vi "PLC-PC.vi"() -> ()   [LabVIEW 2022 SP3]
uses:
  Labview/Globali.vi
panel:
  in  "DB10.DBW 254":u16
  in  "DB10.DBW 252":u16
  in  "DB10.DBW 250":u16
  in  "DB10.DBW 248":u16
  in  "DB10.DBW 246":u16
  in  "DB10.DBW 244":u16
  in  "DB10.DBW 242":u16
  in  "DB10.DBW 240":u16
  in  "DB10.DBW 238":u16
  in  "DB10.DBW 236":u16
  in  "DB10.DBW 234":u16
  in  "DB10.DBW 232":u16
  in  "DB10.DBW 230":u16
  in  "DB10.DBW 228":u16
  in  "DB10.DBW 226":u16
  in  "DB10.DBW 224":u16
  in  "DB10.DBW 222":u16
  in  "DB10.DBW 220":u16
  in  "DB10.DBW 218":u16
  in  "DB10.DBW 216":u16
  in  "DB10.DBW 214":u16
  in  "DB10.DBW 212":u16
  in  "DB10.DBW 210":u16
  in  "DB10.DBW 208":u16
  in  "DB10.DBW 206":u16
  in  "DB10.DBW 204":u16
  in  "DB10.DBW 202":u16
  in  "DB10.DBW 200":u16
  in  "DB10.DBW 198":u16
  in  "DB10.DBW 196":u16
  in  "DB10.DBW 194":u16
  in  "DB10.DBW 192":u16
  in  "DB10.DBW 190":u16
  in  "DB10.DBW 188":u16
  in  "DB10.DBW 186":u16
  in  "DB10.DBW 184":u16
  in  "DB10.DBW 182":u16
  in  "DB10.DBW 180":u16
  in  "DB10.DBW 178":u16
  in  "DB10.DBW 176":u16
  in  "DB10.DBW 174":u16
  in  "DB10.DBW 172":u16
  in  "DB10.DBW 170":u16
  in  "DB10.DBW 168":u16
  in  "DB10.DBW 166":u16
  in  "DB10.DBW 164":u16
  in  "DB10.DBW 162":u16
  in  "DB10.DBW 160":u16
  in  "DB10.DBW 158":u16
  in  "DB10.DBW 156":u16
  in  "DB10.DBW 154":u16
  in  "DB10.DBW 152":u16
  in  "DB10.DBW 150":u16
  in  "DB10.DBW 148":u16
  in  "DB10.DBW 146":u16
  in  "DB10.DBW 144":u16
  in  "DB10.DBW 142":u16
  in  "DB10.DBW 140":u16
  in  "DB10.DBW 138":u16
  in  "DB10.DBW 136":u16
  in  "DB10.DBW 134":u16
  in  "DB10.DBW 132":u16
  in  "DB10.DBW 130":u16
  in  "DB10.DBW 128":u16
  in  "DB10.DBW 126":u16
  in  "DB10.DBW 124":u16
  in  "DB10.DBW 122":u16
  in  "DB10.DBW 120":u16
  in  "DB10.DBW 118":u16
  in  "DB10.DBW 116":u16
  in  "DB10.DBW 114":u16
  in  "DB10.DBW 112":u16
  in  "DB10.DBW 110":u16
  in  "DB10.DBW 108":u16
  in  "DB10.DBW 106":u16
  in  "DB10.DBW 104":u16
  in  "DB10.DBW 102":u16
  in  "DB10.DBW 100":u16
  in  "DB10.DBW 98":u16
  in  "DB10.DBW 96":u16
  in  "DB10.DBW 94":u16
  in  "DB10.DBW 92":u16
  in  "DB10.DBW 90":u16
  in  "DB10.DBW 88":u16
  in  "DB10.DBW 86":u16
  in  "DB10.DBW 84":u16
  in  "DB10.DBW 82":u16
  in  "DB10.DBW 80":u16
  in  "DB10.DBW 78":u16
  in  "DB10.DBW 76":u16
  in  "DB10.DBW 74":u16
  in  "DB10.DBW 72":u16
  in  "DB10.DBW 70":u16
  in  "DB10.DBW 68":u16
  in  "DB10.DBW 66":u16
  in  "DB10.DBW 64":u16
  in  "DB10.DBW 62":u16
  in  "DB10.DBW 60":u16
  in  "DB10.DBW 58":u16
  in  "DB10.DBW 56":u16
  in  "DB10.DBW 54":u16
  in  "DB10.DBW 52":u16
  in  "DB10.DBW 50":u16
  in  "DB10.DBW 48":u16
  in  "DB10.DBW 46":u16
  in  "DB10.DBW 44":u16
  in  "DB10.DBW 42":u16
  in  "DB10.DBW 40":u16
  in  "DB10.DBW 38":u16
  in  "DB10.DBW 36":u16
  in  "DB10.DBW 34":u16
  in  "DB10.DBW 32":u16
  in  "DB10.DBW 30":u16
  in  "DB10.DBW 28":u16
  in  "DB10.DBW 26":u16
  in  "DB10.DBW 24":u16
  in  "DB10.DBW 22":u16
  in  "DB10.DBW 20":u16
  in  "DB10.DBW 18":u16
  in  "DB10.DBW 16":u16
  in  "DB10.DBW 14":u16
  in  "DB10.DBW 12":u16
  in  "DB10.DBW 10":u16
  in  "DB10.DBW 8":u16
  in  "DB10.DBW 6":u16
  in  "DB10.DBW 4":u16
  in  "DB10.DBW 2":u16
  in  "DB10.DBW 0":u16
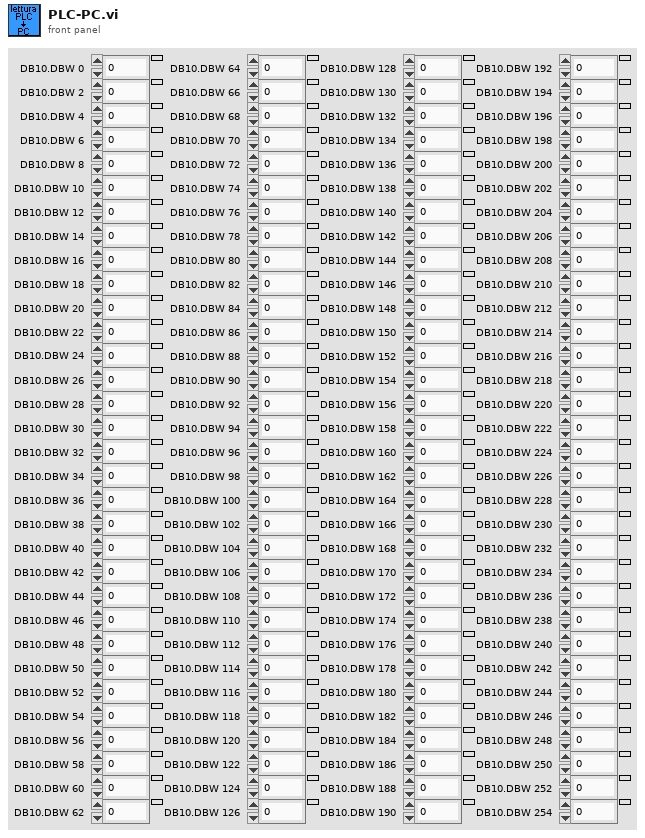
[diagram p1: front panel]
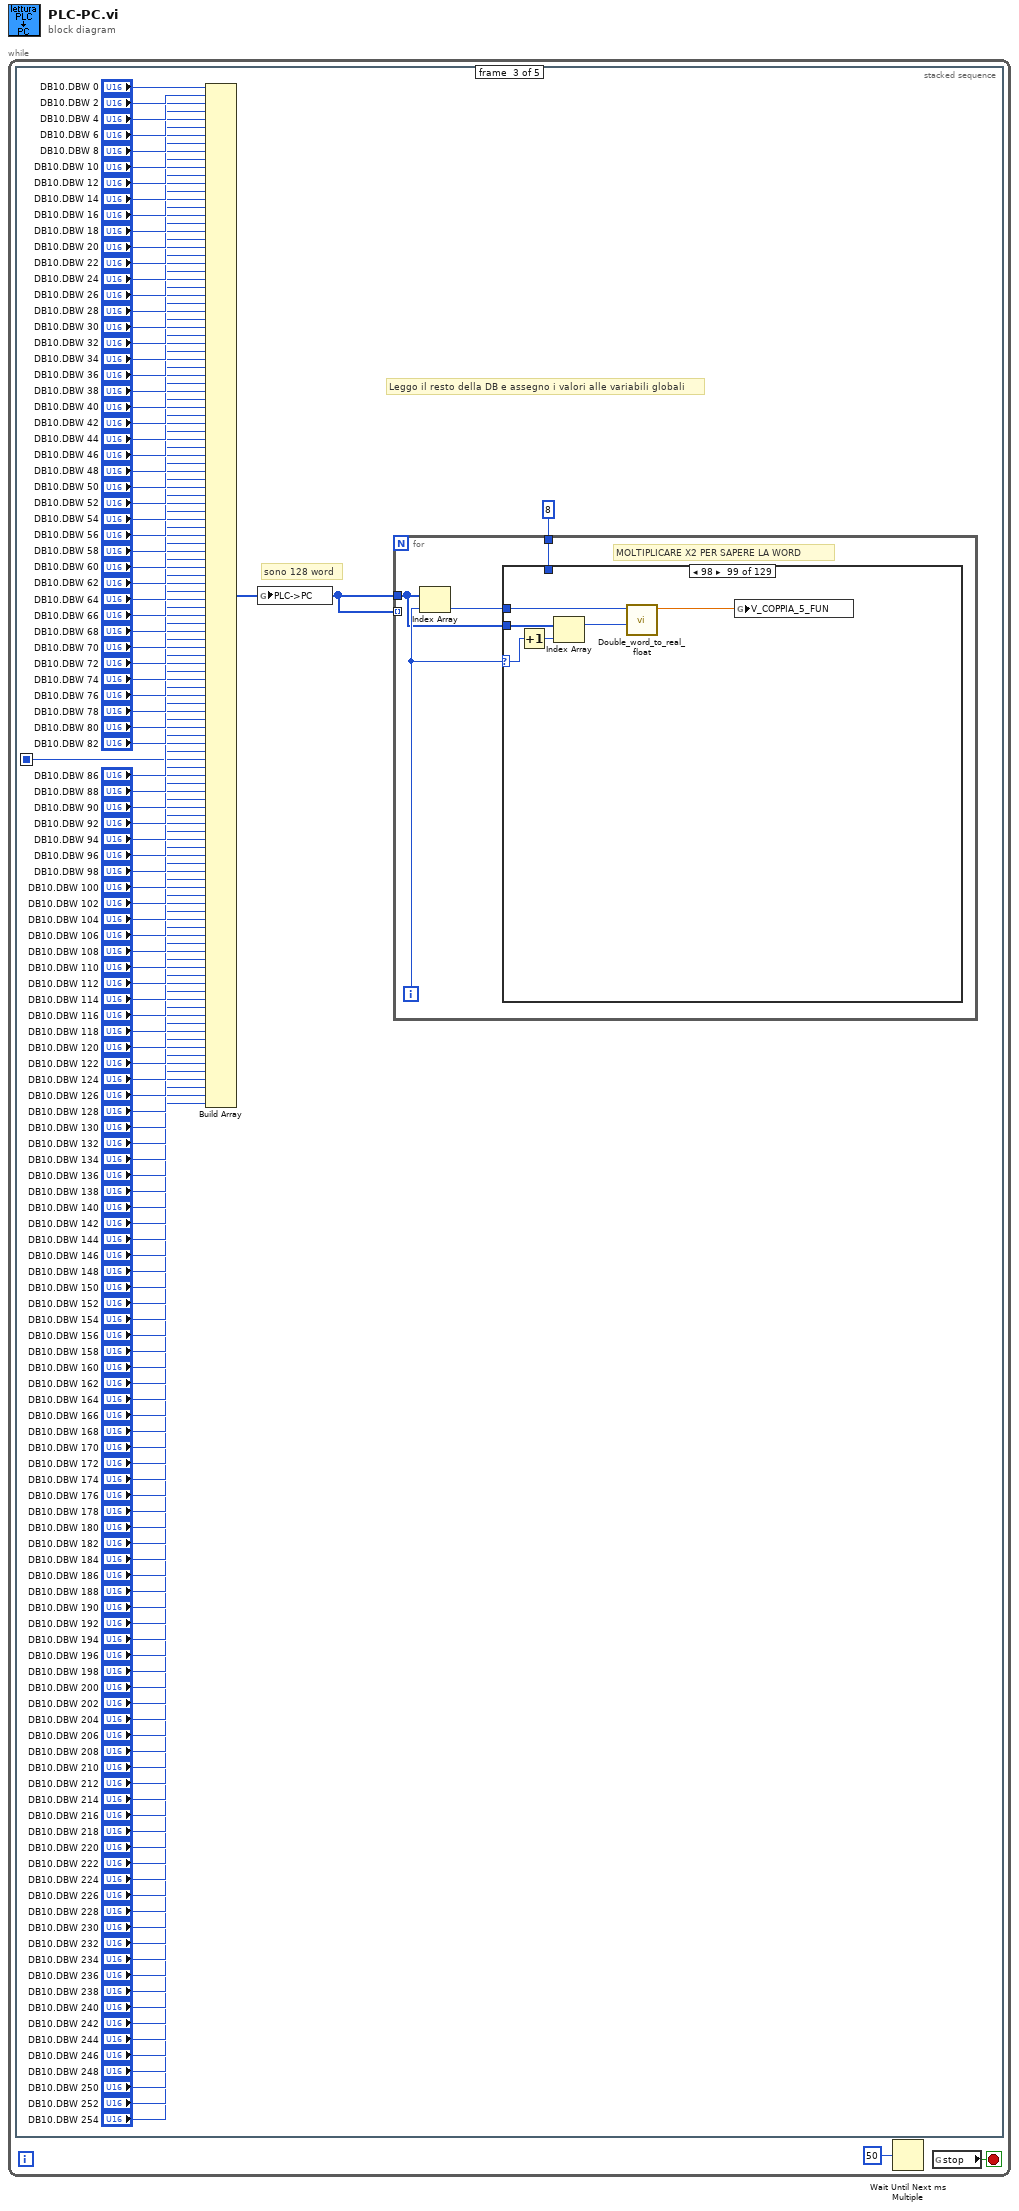
[diagram p0: block diagram]
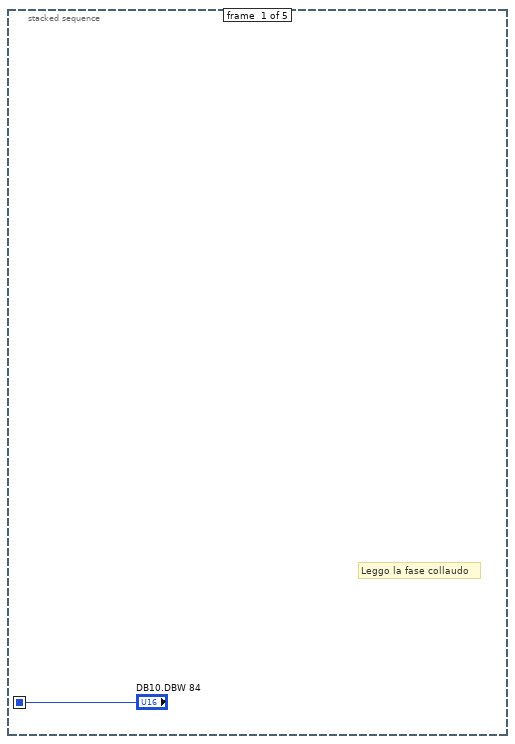
[diagram p2: hidden frame]
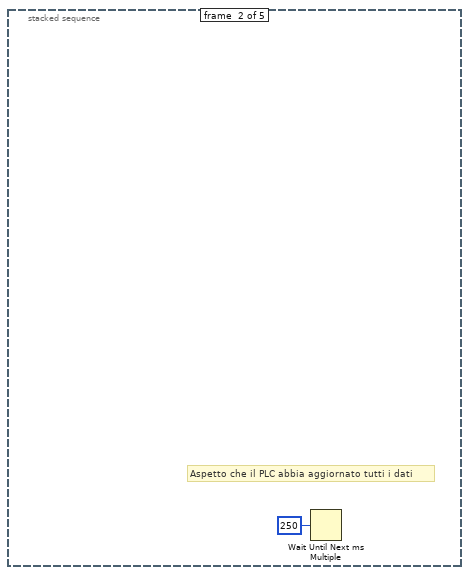
[diagram p3: hidden frame]
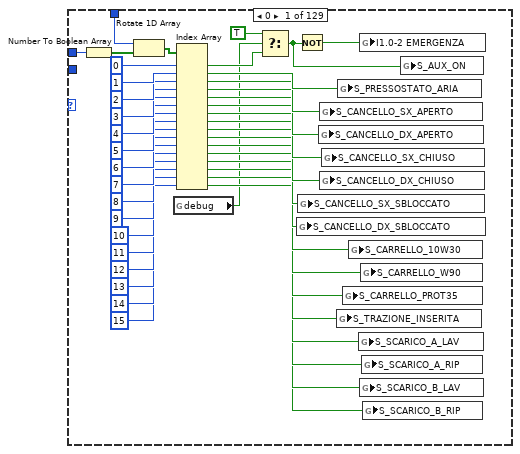
[diagram p4: hidden frame]
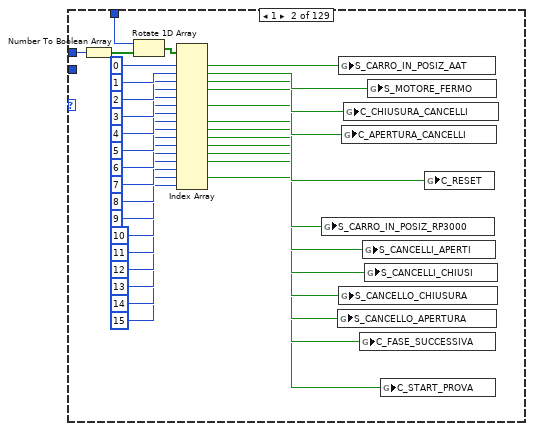
[diagram p5: hidden frame]
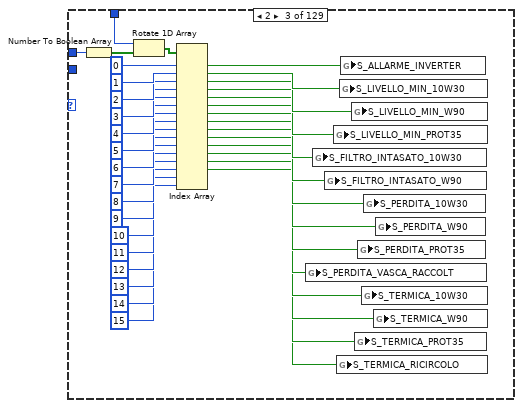
[diagram p6: hidden frame]
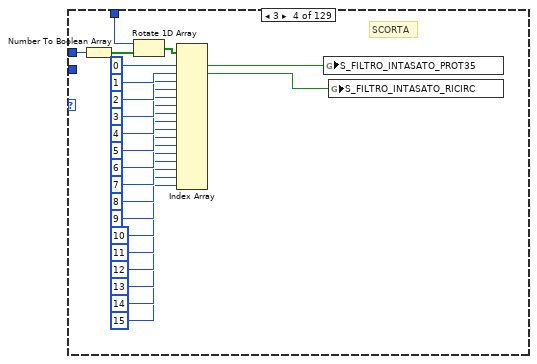
[diagram p7: hidden frame]
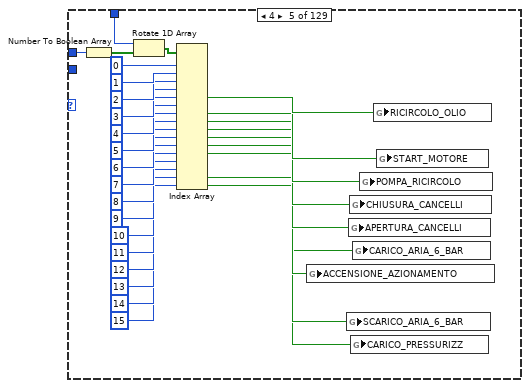
[diagram p8: hidden frame]
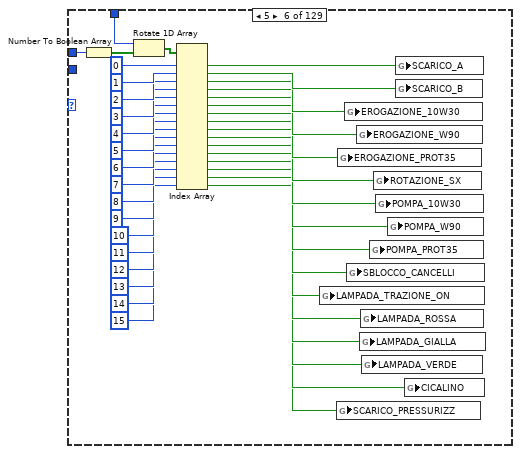
[diagram p9: hidden frame]
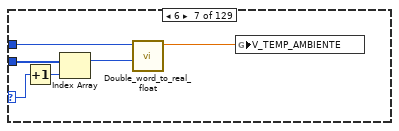
[diagram p10: hidden frame]
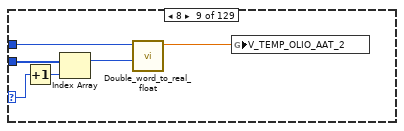
[diagram p12: hidden frame]
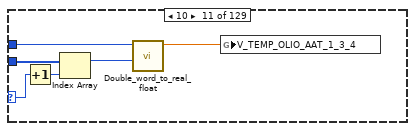
[diagram p14: hidden frame]
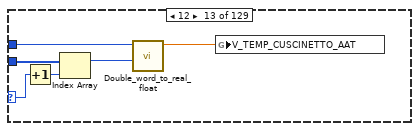
[diagram p16: hidden frame]
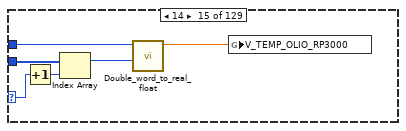
[diagram p18: hidden frame]
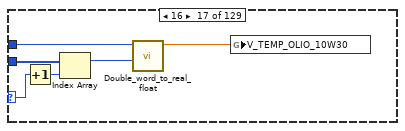
[diagram p20: hidden frame]
diagram:
  n1 = while {
    stop <- w1 stop-if-true
    n2 = stacked-sequence {
      seq-local: ["DB10.DBW 84" _ _ _ _] -> [_ _ w5 _ w990]
      frame #0 {
        # "Leggo la fase collaudo"
      }
      frame #1 {
        # "Aspetto che il PLC abbia aggiornato tutti i dati"
        n3 = Wait Until Next ms Multiple(millisecond multiple=u32 250) -> ()  [unwired: 1 out]
      }
      frame #2 {
        # "Leggo il resto della DB e assegno i valori alle variabili globali"
        # "sono 128 word"
        n4 = Build Array("DB10.DBW 0", "DB10.DBW 2", "DB10.DBW 4", "DB10.DBW 6", "DB10.DBW 8", "DB10.DBW 10", "DB10.DBW 12", "DB10.DBW 14", "DB10.DBW 16", "DB10.DBW 18", "DB10.DBW 20", "DB10.DBW 22", "DB10.DBW 24", "DB10.DBW 26", "DB10.DBW 28", "DB10.DBW 30", "DB10.DBW 32", "DB10.DBW 34", "DB10.DBW 36", "DB10.DBW 38", "DB10.DBW 40", "DB10.DBW 42", "DB10.DBW 44", "DB10.DBW 46", "DB10.DBW 48", "DB10.DBW 50", "DB10.DBW 52", "DB10.DBW 54", "DB10.DBW 56", "DB10.DBW 58", "DB10.DBW 60", "DB10.DBW 62", "DB10.DBW 64", "DB10.DBW 66", "DB10.DBW 68", "DB10.DBW 70", "DB10.DBW 72", "DB10.DBW 74", "DB10.DBW 76", "DB10.DBW 78", "DB10.DBW 80", "DB10.DBW 82", w5, "DB10.DBW 86", "DB10.DBW 88", "DB10.DBW 90", "DB10.DBW 92", "DB10.DBW 94", "DB10.DBW 96", "DB10.DBW 98", "DB10.DBW 100", "DB10.DBW 102", "DB10.DBW 104", "DB10.DBW 106", "DB10.DBW 108", "DB10.DBW 110", "DB10.DBW 112", "DB10.DBW 114", "DB10.DBW 116", "DB10.DBW 118", "DB10.DBW 120", "DB10.DBW 122", "DB10.DBW 124", "DB10.DBW 126", "DB10.DBW 128", "DB10.DBW 130", "DB10.DBW 132", "DB10.DBW 134", "DB10.DBW 136", "DB10.DBW 138", "DB10.DBW 140", "DB10.DBW 142", "DB10.DBW 144", "DB10.DBW 146", "DB10.DBW 148", "DB10.DBW 150", "DB10.DBW 152", "DB10.DBW 154", "DB10.DBW 156", "DB10.DBW 158", "DB10.DBW 160", "DB10.DBW 162", "DB10.DBW 164", "DB10.DBW 166", "DB10.DBW 168", "DB10.DBW 170", "DB10.DBW 172", "DB10.DBW 174", "DB10.DBW 176", "DB10.DBW 178", "DB10.DBW 180", "DB10.DBW 182", "DB10.DBW 184", "DB10.DBW 186", "DB10.DBW 188", "DB10.DBW 190", "DB10.DBW 192", "DB10.DBW 194", "DB10.DBW 196", "DB10.DBW 198", "DB10.DBW 200", "DB10.DBW 202", "DB10.DBW 204", "DB10.DBW 206", "DB10.DBW 208", "DB10.DBW 210", "DB10.DBW 212", "DB10.DBW 214", "DB10.DBW 216", "DB10.DBW 218", "DB10.DBW 220", "DB10.DBW 222", "DB10.DBW 224", "DB10.DBW 226", "DB10.DBW 228", "DB10.DBW 230", "DB10.DBW 232", "DB10.DBW 234", "DB10.DBW 236", "DB10.DBW 238", "DB10.DBW 240", "DB10.DBW 242", "DB10.DBW 244", "DB10.DBW 246", "DB10.DBW 248", "DB10.DBW 250", "DB10.DBW 252", "DB10.DBW 254") -> (w6:u16[])
        n5 = global write "Globali.vi" "PLC->PC"(w6) -> ()
        n6 = for {
          tunnel: w6 -> [w136]
          tunnel: w6 -> [_] mode=indexing
          tunnel: 8 ("n") -> [w135]
          i -> [w138]
          # "MOLTIPLICARE X2 PER SAPERE LA WORD"
          n7 = Index Array(array=w136, index=w138) -> (element=w137:u16)
          n8 = case shown="98" w138 {
            selector: w138 -> [_ _ _ _ _ _ w335 _ w341 _ w347 _ w353 _ w359 _ w365 _ w371 _ w376 _ w382 _ w388 _ w394 _ w400 _ w406 _ _ _ _ _ w415 _ _ _ _ _ _ _ w472 _ _ w499 _ w505 _ _ w532 _ w538 _ _ w565 _ w571 _ w577 _ _ w604 _ w610 _ _ w637 _ w643 _ w649 _ _ w676 _ w682 _ _ w709 _ _ w738 _ w744 _ _ w771 _ w777 _ _ w804 _ w810 _ w816 _ _ w843 _ w849 _ _ w876 _ _ w903 _ _ w930 _ w934 _ w940 _ w946 _ w952 _ w958 _ _ _ _ _ _]
            tunnel: w137 -> [w178 w210 w244 w266 w295 w331 w333 _ w339 _ w345 _ w351 _ w357 _ w363 _ w369 _ w374 _ w380 _ w386 _ w392 _ w398 _ w404 _ w409 w410 w411 _ w413 _ w440 w441 w442 w443 _ w468 w470 _ w495 w497 _ w503 _ w528 w530 _ w536 _ w561 w563 _ w569 _ w575 _ w600 w602 _ w608 _ w633 w635 _ w641 _ w647 _ w672 w674 _ w680 _ w705 w707 _ w734 w736 _ w742 _ w767 w769 _ w775 _ w800 w802 _ w808 _ w814 _ w839 w841 _ w847 _ w872 w874 _ w899 w901 _ w927 w928 _ w936 _ w942 _ w948 _ w954 _ w960 _ w968 w988 _ _ _]
            tunnel: w136 -> [_ _ _ _ _ _ w337 _ w343 _ w349 _ w355 _ w361 _ w367 _ w373 _ w378 _ w384 _ w390 _ w396 _ w402 _ w408 _ _ _ _ _ w417 _ _ _ _ _ _ _ w474 _ _ w501 _ w507 _ _ w534 _ w540 _ _ w567 _ w573 _ w579 _ _ w606 _ w612 _ _ w639 _ w645 _ w651 _ _ w678 _ w684 _ _ w711 _ _ w740 _ w746 _ _ w773 _ w779 _ _ w806 _ w812 _ w818 _ _ w845 _ w851 _ _ w878 _ _ w905 _ _ w929 _ w935 _ w941 _ w947 _ w953 _ w959 _ _ _ _ _ _]
            tunnel: w135 -> [w144 w186 w211 w247 w271 w297 _ _ _ _ _ _ _ _ _ _ _ _ _ _ _ _ _ _ _ _ _ _ _ _ _ _ _ _ _ _ _ _ w419 _ _ _ _ w444 _ _ w475 _ _ _ _ w508 _ _ _ _ w541 _ _ _ _ _ _ w580 _ _ _ _ w613 _ _ _ _ _ _ w652 _ _ _ _ w685 _ _ w712 _ _ _ _ w747 _ _ _ _ w780 _ _ _ _ _ _ w819 _ _ _ _ w852 _ _ w879 _ _ w906 _ _ _ _ _ _ _ _ _ _ _ _ w967 _ _ _ _]
            frame 0 {
              n9 = Number To Boolean Array(number=w178) -> (Boolean array=w177:bool[])
              n10 = Rotate 1D Array(1:w177, 2:w144) -> (0:w145:bool[])
              n11 = global read "Globali.vi" "debug"() -> (w142:bool)
              n12 = Index Array(array=w145, index #1=0 ("index"), index #2=1 ("index"), index #3=2 ("index"), index #4=3 ("index"), index #5=4 ("index"), index #6=5 ("index"), index #7=6 ("index"), index #8=7 ("index"), index #9=8 ("index"), index #10=9 ("index"), index #11=10 ("index"), index #12=11 ("index"), index #13=12 ("index"), index #14=13 ("index"), index #15=14 ("index"), index #16=15 ("index")) -> (element #1=w143:bool, element #2=w160:bool, element #3=w159:bool, element #4=w158:bool, element #5=w157:bool, element #6=w156:bool, element #7=w155:bool, element #8=w154:bool, element #9=w153:bool, element #10=w152:bool, element #11=w151:bool, element #12=w150:bool, element #13=w149:bool, element #14=w148:bool, element #15=w147:bool, element #16=w146:bool)
              n13 = Select(t=TRUE, s=w142, f=w143) -> (s? t:f=w140:bool)
              n14 = Not(x=w140) -> (.not. x?=w139:bool)
              n15 = global write "Globali.vi" "S_CANCELLO_DX_SBLOCCATO"(w154) -> ()
              n16 = global write "Globali.vi" "S_CANCELLO_SX_SBLOCCATO"(w155) -> ()
              n17 = global write "Globali.vi" "S_CANCELLO_DX_APERTO"(w158) -> ()
              n18 = global write "Globali.vi" "S_CANCELLO_SX_APERTO"(w159) -> ()
              n19 = global write "Globali.vi" "S_CANCELLO_DX_CHIUSO"(w156) -> ()
              n20 = global write "Globali.vi" "S_CANCELLO_SX_CHIUSO"(w157) -> ()
              n21 = global write "Globali.vi" "S_TRAZIONE_INSERITA"(w150) -> ()
              n22 = global write "Globali.vi" "S_PRESSOSTATO_ARIA"(w160) -> ()
              n23 = global write "Globali.vi" "S_CARRELLO_PROT35"(w151) -> ()
              n24 = global write "Globali.vi" "S_CARRELLO_10W30"(w153) -> ()
              n25 = global write "Globali.vi" "S_SCARICO_A_LAV"(w149) -> ()
              n26 = global write "Globali.vi" "I1.0-2 EMERGENZA"(w139) -> ()
              n27 = global write "Globali.vi" "S_SCARICO_B_LAV"(w147) -> ()
              n28 = global write "Globali.vi" "S_CARRELLO_W90"(w152) -> ()
              n29 = global write "Globali.vi" "S_SCARICO_A_RIP"(w148) -> ()
              n30 = global write "Globali.vi" "S_SCARICO_B_RIP"(w146) -> ()
              n31 = global write "Globali.vi" "S_AUX_ON"(w140) -> ()
            }
            frame 1 {
              n32 = Number To Boolean Array(number=w210) -> (Boolean array=w209:bool[])
              n33 = Rotate 1D Array(1:w209, 2:w186) -> (0:w187:bool[])
              n34 = Index Array(array=w187, index #1=0 ("index"), index #2=1 ("index"), index #3=2 ("index"), index #4=3 ("index"), index #5=4 ("index"), index #6=5 ("index"), index #7=6 ("index"), index #8=7 ("index"), index #9=8 ("index"), index #10=9 ("index"), index #11=10 ("index"), index #12=11 ("index"), index #13=12 ("index"), index #14=13 ("index"), index #15=14 ("index"), index #16=15 ("index")) -> (element #1=w192:bool, element #2=w191:bool, element #3=w190:bool, element #4=w189:bool, element #6=w188:bool, element #8=w185:bool, element #9=w184:bool, element #10=w183:bool, element #11=w182:bool, element #12=w181:bool, element #13=w180:bool, element #15=w179:bool)  [unwired: 4 out]
              n35 = global write "Globali.vi" "S_CARRO_IN_POSIZ_RP3000"(w185) -> ()
              n36 = global write "Globali.vi" "S_CANCELLO_APERTURA"(w181) -> ()
              n37 = global write "Globali.vi" "S_CARRO_IN_POSIZ_AAT"(w192) -> ()
              n38 = global write "Globali.vi" "S_CANCELLO_CHIUSURA"(w182) -> ()
              n39 = global write "Globali.vi" "C_APERTURA_CANCELLI"(w189) -> ()
              n40 = global write "Globali.vi" "C_CHIUSURA_CANCELLI"(w190) -> ()
              n41 = global write "Globali.vi" "C_FASE_SUCCESSIVA"(w180) -> ()
              n42 = global write "Globali.vi" "S_CANCELLI_APERTI"(w184) -> ()
              n43 = global write "Globali.vi" "S_CANCELLI_CHIUSI"(w183) -> ()
              n44 = global write "Globali.vi" "S_MOTORE_FERMO"(w191) -> ()
              n45 = global write "Globali.vi" "C_START_PROVA"(w179) -> ()
              n46 = global write "Globali.vi" "C_RESET"(w188) -> ()
            }
            frame 2 {
              n47 = Number To Boolean Array(number=w244) -> (Boolean array=w243:bool[])
              n48 = Rotate 1D Array(1:w243, 2:w211) -> (0:w212:bool[])
              n49 = Index Array(array=w212, index #1=0 ("index"), index #2=1 ("index"), index #3=2 ("index"), index #4=3 ("index"), index #5=4 ("index"), index #6=5 ("index"), index #7=6 ("index"), index #8=7 ("index"), index #9=8 ("index"), index #10=9 ("index"), index #11=10 ("index"), index #12=11 ("index"), index #13=12 ("index"), index #14=13 ("index"), index #15=14 ("index"), index #16=15 ("index")) -> (element #1=w226:bool, element #2=w225:bool, element #3=w224:bool, element #4=w223:bool, element #5=w222:bool, element #6=w221:bool, element #7=w220:bool, element #8=w219:bool, element #9=w218:bool, element #10=w217:bool, element #11=w216:bool, element #12=w215:bool, element #13=w214:bool, element #14=w213:bool)  [unwired: 2 out]
              n50 = global write "Globali.vi" "S_PERDITA_VASCA_RACCOLT"(w217) -> ()
              n51 = global write "Globali.vi" "S_FILTRO_INTASATO_10W30"(w222) -> ()
              n52 = global write "Globali.vi" "S_FILTRO_INTASATO_W90"(w221) -> ()
              n53 = global write "Globali.vi" "S_LIVELLO_MIN_PROT35"(w223) -> ()
              n54 = global write "Globali.vi" "S_TERMICA_RICIRCOLO"(w213) -> ()
              n55 = global write "Globali.vi" "S_LIVELLO_MIN_10W30"(w225) -> ()
              n56 = global write "Globali.vi" "S_ALLARME_INVERTER"(w226) -> ()
              n57 = global write "Globali.vi" "S_LIVELLO_MIN_W90"(w224) -> ()
              n58 = global write "Globali.vi" "S_TERMICA_PROT35"(w214) -> ()
              n59 = global write "Globali.vi" "S_PERDITA_PROT35"(w218) -> ()
              n60 = global write "Globali.vi" "S_TERMICA_10W30"(w216) -> ()
              n61 = global write "Globali.vi" "S_PERDITA_10W30"(w220) -> ()
              n62 = global write "Globali.vi" "S_TERMICA_W90"(w215) -> ()
              n63 = global write "Globali.vi" "S_PERDITA_W90"(w219) -> ()
            }
            frame 3 {
              # "SCORTA"
              n64 = Number To Boolean Array(number=w266) -> (Boolean array=w265:bool[])
              n65 = Rotate 1D Array(1:w265, 2:w247) -> (0:w248:bool[])
              n66 = Index Array(array=w248, index #1=0 ("index"), index #2=1 ("index"), index #3=2 ("index"), index #4=3 ("index"), index #5=4 ("index"), index #6=5 ("index"), index #7=6 ("index"), index #8=7 ("index"), index #9=8 ("index"), index #10=9 ("index"), index #11=10 ("index"), index #12=11 ("index"), index #13=12 ("index"), index #14=13 ("index"), index #15=14 ("index"), index #16=15 ("index")) -> (element #1=w246:bool, element #2=w245:bool)  [unwired: 14 out]
              n67 = global write "Globali.vi" "S_FILTRO_INTASATO_PROT35"(w246) -> ()
              n68 = global write "Globali.vi" "S_FILTRO_INTASATO_RICIRC"(w245) -> ()
            }
            frame 4 {
              n69 = Number To Boolean Array(number=w295) -> (Boolean array=w294:bool[])
              n70 = Rotate 1D Array(1:w294, 2:w271) -> (0:w272:bool[])
              n71 = Index Array(array=w272, index #1=0 ("index"), index #2=1 ("index"), index #3=2 ("index"), index #4=3 ("index"), index #5=4 ("index"), index #6=5 ("index"), index #7=6 ("index"), index #8=7 ("index"), index #9=8 ("index"), index #10=9 ("index"), index #11=10 ("index"), index #12=11 ("index"), index #13=12 ("index"), index #14=13 ("index"), index #15=14 ("index"), index #16=15 ("index")) -> (element #5=w277:bool, element #7=w276:bool, element #8=w275:bool, element #9=w274:bool, element #10=w273:bool, element #11=w269:bool, element #12=w270:bool, element #15=w268:bool, element #16=w267:bool)  [unwired: 7 out]
              n72 = global write "Globali.vi" "ACCENSIONE_AZIONAMENTO"(w270) -> ()
              n73 = global write "Globali.vi" "SCARICO_ARIA_6_BAR"(w268) -> ()
              n74 = global write "Globali.vi" "APERTURA_CANCELLI"(w273) -> ()
              n75 = global write "Globali.vi" "CHIUSURA_CANCELLI"(w274) -> ()
              n76 = global write "Globali.vi" "CARICO_PRESSURIZZ"(w267) -> ()
              n77 = global write "Globali.vi" "CARICO_ARIA_6_BAR"(w269) -> ()
              n78 = global write "Globali.vi" "POMPA_RICIRCOLO"(w275) -> ()
              n79 = global write "Globali.vi" "RICIRCOLO_OLIO"(w277) -> ()
              n80 = global write "Globali.vi" "START_MOTORE"(w276) -> ()
            }
            frame 5 {
              n81 = Number To Boolean Array(number=w331) -> (Boolean array=w330:bool[])
              n82 = Rotate 1D Array(1:w330, 2:w297) -> (0:w298:bool[])
              n83 = Index Array(array=w298, index #1=0 ("index"), index #2=1 ("index"), index #3=2 ("index"), index #4=3 ("index"), index #5=4 ("index"), index #6=5 ("index"), index #7=6 ("index"), index #8=7 ("index"), index #9=8 ("index"), index #10=9 ("index"), index #11=10 ("index"), index #12=11 ("index"), index #13=12 ("index"), index #14=13 ("index"), index #15=14 ("index"), index #16=15 ("index")) -> (element #1=w313:bool, element #2=w312:bool, element #3=w311:bool, element #4=w310:bool, element #5=w309:bool, element #6=w308:bool, element #7=w307:bool, element #8=w306:bool, element #9=w305:bool, element #10=w304:bool, element #11=w303:bool, element #12=w302:bool, element #13=w301:bool, element #14=w300:bool, element #15=w299:bool, element #16=w296:bool)
              n84 = global write "Globali.vi" "LAMPADA_TRAZIONE_ON"(w303) -> ()
              n85 = global write "Globali.vi" "SCARICO_PRESSURIZZ"(w296) -> ()
              n86 = global write "Globali.vi" "EROGAZIONE_PROT35"(w309) -> ()
              n87 = global write "Globali.vi" "EROGAZIONE_10W30"(w311) -> ()
              n88 = global write "Globali.vi" "SBLOCCO_CANCELLI"(w304) -> ()
              n89 = global write "Globali.vi" "EROGAZIONE_W90"(w310) -> ()
              n90 = global write "Globali.vi" "LAMPADA_GIALLA"(w301) -> ()
              n91 = global write "Globali.vi" "LAMPADA_ROSSA"(w302) -> ()
              n92 = global write "Globali.vi" "LAMPADA_VERDE"(w300) -> ()
              n93 = global write "Globali.vi" "POMPA_PROT35"(w305) -> ()
              n94 = global write "Globali.vi" "ROTAZIONE_SX"(w308) -> ()
              n95 = global write "Globali.vi" "POMPA_10W30"(w307) -> ()
              n96 = global write "Globali.vi" "POMPA_W90"(w306) -> ()
              n97 = global write "Globali.vi" "SCARICO_A"(w313) -> ()
              n98 = global write "Globali.vi" "SCARICO_B"(w312) -> ()
              n99 = global write "Globali.vi" "CICALINO"(w299) -> ()
            }
            frame 6 {
              n100 = Increment(x=w335) -> (x+1=w336:i32)
              n101 = Index Array(array=w337, index=w336) -> (element=w334:u16)
              n102 = call "Double_word_to_real_float.vi"("Seconda WORD"=w334, "Prima WORD"=w333) -> ("Real float"=w332:dbl)  [unwired: 9 in]
              n103 = global write "Globali.vi" "V_TEMP_AMBIENTE"(w332) -> ()
            }
            frame 7 {
            }
            frame 8 {
              n104 = Increment(x=w341) -> (x+1=w342:i32)
              n105 = Index Array(array=w343, index=w342) -> (element=w340:u16)
              n106 = call "Double_word_to_real_float.vi"("Seconda WORD"=w340, "Prima WORD"=w339) -> ("Real float"=w338:dbl)  [unwired: 9 in]
              n107 = global write "Globali.vi" "V_TEMP_OLIO_AAT_2"(w338) -> ()
            }
            frame 9 {
            }
            frame 10 {
              n108 = Increment(x=w347) -> (x+1=w348:i32)
              n109 = Index Array(array=w349, index=w348) -> (element=w346:u16)
              n110 = call "Double_word_to_real_float.vi"("Seconda WORD"=w346, "Prima WORD"=w345) -> ("Real float"=w344:dbl)  [unwired: 9 in]
              n111 = global write "Globali.vi" "V_TEMP_OLIO_AAT_1_3_4"(w344) -> ()
            }
            frame 11 {
            }
            frame 12 {
              n112 = Increment(x=w353) -> (x+1=w354:i32)
              n113 = Index Array(array=w355, index=w354) -> (element=w352:u16)
              n114 = call "Double_word_to_real_float.vi"("Seconda WORD"=w352, "Prima WORD"=w351) -> ("Real float"=w350:dbl)  [unwired: 9 in]
              n115 = global write "Globali.vi" "V_TEMP_CUSCINETTO_AAT"(w350) -> ()
            }
            frame 13 {
            }
            frame 14 {
              n116 = Increment(x=w359) -> (x+1=w360:i32)
              n117 = Index Array(array=w361, index=w360) -> (element=w358:u16)
              n118 = call "Double_word_to_real_float.vi"("Seconda WORD"=w358, "Prima WORD"=w357) -> ("Real float"=w356:dbl)  [unwired: 9 in]
              n119 = global write "Globali.vi" "V_TEMP_OLIO_RP3000"(w356) -> ()
            }
            frame 15 {
            }
            frame 16 {
              n120 = Increment(x=w365) -> (x+1=w366:i32)
              n121 = Index Array(array=w367, index=w366) -> (element=w364:u16)
              n122 = call "Double_word_to_real_float.vi"("Seconda WORD"=w364, "Prima WORD"=w363) -> ("Real float"=w362:dbl)  [unwired: 9 in]
              n123 = global write "Globali.vi" "V_TEMP_OLIO_10W30"(w362) -> ()
            }
            frame 17 {
            }
            frame 18 {
              n124 = Increment(x=w371) -> (x+1=w372:i32)
              n125 = Index Array(array=w373, index=w372) -> (element=w370:u16)
              n126 = call "Double_word_to_real_float.vi"("Seconda WORD"=w370, "Prima WORD"=w369) -> ("Real float"=w368:dbl)  [unwired: 9 in]
              n127 = global write "Globali.vi" "V_TEMP_OLIO_10W90"(w368) -> ()
            }
            frame 19 {
            }
            frame 20 {
              # "SCORTA"
              n128 = Increment(x=w376) -> (x+1=w377:i32)
              n129 = Index Array(array=w378, index=w377) -> (element=w375:u16)
              n130 = call "Double_word_to_real_float.vi"("Seconda WORD"=w375, "Prima WORD"=w374) -> ()  [unwired: 9 in, 1 out]
            }
            frame 21 {
            }
            frame 22 {
              n131 = Increment(x=w382) -> (x+1=w383:i32)
              n132 = Index Array(array=w384, index=w383) -> (element=w381:u16)
              n133 = call "Double_word_to_real_float.vi"("Seconda WORD"=w381, "Prima WORD"=w380) -> ("Real float"=w379:dbl)  [unwired: 9 in]
              n134 = global write "Globali.vi" "V_PRESS_ARIA_6_BAR"(w379) -> ()
            }
            frame 23 {
            }
            frame 24 {
              n135 = Increment(x=w388) -> (x+1=w389:i32)
              n136 = Index Array(array=w390, index=w389) -> (element=w387:u16)
              n137 = call "Double_word_to_real_float.vi"("Seconda WORD"=w387, "Prima WORD"=w386) -> ("Real float"=w385:dbl)  [unwired: 9 in]
              n138 = global write "Globali.vi" "V_PRESSURIZZAZIONE"(w385) -> ()
            }
            frame 25 {
            }
            frame 26 {
              n139 = Increment(x=w394) -> (x+1=w395:i32)
              n140 = Index Array(array=w396, index=w395) -> (element=w393:u16)
              n141 = call "Double_word_to_real_float.vi"("Seconda WORD"=w393, "Prima WORD"=w392) -> ("Real float"=w391:dbl)  [unwired: 9 in]
              n142 = global write "Globali.vi" "V_PRESS_OLIO_RICIRCOLO"(w391) -> ()
            }
            frame 27 {
            }
            frame 28 {
              n143 = Increment(x=w400) -> (x+1=w401:i32)
              n144 = Index Array(array=w402, index=w401) -> (element=w399:u16)
              n145 = call "Double_word_to_real_float.vi"("Seconda WORD"=w399, "Prima WORD"=w398) -> ("Real float"=w397:dbl)  [unwired: 9 in]
              n146 = global write "Globali.vi" "V_PORTATA_RICIRCOLO"(w397) -> ()
            }
            frame 29 {
            }
            frame 30 {
              n147 = Increment(x=w406) -> (x+1=w407:i32)
              n148 = Index Array(array=w408, index=w407) -> (element=w405:u16)
              n149 = call "Double_word_to_real_float.vi"("Seconda WORD"=w405, "Prima WORD"=w404) -> ("Real float"=w403:dbl)  [unwired: 9 in]
              n150 = global write "Globali.vi" "V_COPPIA_ASSE_TRASCINAM"(w403) -> ()
            }
            frame 31 {
            }
            frame 32 {
              n151 = global write "Globali.vi" "VI_VEL_MOT"(w409) -> ()
            }
            frame 33 {
              n152 = global write "Globali.vi" "VO_VEL_MOT"(w410) -> ()
            }
            frame 34 {
              n153 = global write "Globali.vi" "VI_COPPIA_MOT"(w411) -> ()
            }
            frame 35 {
            }
            frame 36 {
              n154 = Increment(x=w415) -> (x+1=w416:i32)
              n155 = Index Array(array=w417, index=w416) -> (element=w414:u16)
              n156 = call "Double_word_to_real_float.vi"("Seconda WORD"=w414, "Prima WORD"=w413) -> ("Real float"=w412:dbl)  [unwired: 9 in]
              n157 = global write "Globali.vi" "V_GONFIAGGIO_STAB"(w412) -> ()
            }
            frame 37 {
            }
            frame 38 {
              n158 = Number To Boolean Array(number=w440) -> (Boolean array=w439:bool[])
              n159 = Rotate 1D Array(1:w439, 2:w419) -> (0:w420:bool[])
              n160 = Index Array(array=w420, index #1=0 ("index"), index #2=1 ("index"), index #3=2 ("index"), index #4=3 ("index"), index #5=4 ("index"), index #6=5 ("index"), index #7=6 ("index"), index #8=7 ("index"), index #9=8 ("index"), index #10=9 ("index"), index #11=10 ("index"), index #12=11 ("index"), index #13=12 ("index"), index #14=13 ("index"), index #15=14 ("index"), index #16=15 ("index")) -> (element #1=w422:bool, element #2=w421:bool, element #3=w418:bool)  [unwired: 13 out]
              n161 = global write "Globali.vi" "S_ALLARME"(w418) -> ()
              n162 = global write "Globali.vi" "S_AUTO"(w421) -> ()
              n163 = global write "Globali.vi" "S_MAN"(w422) -> ()
            }
            frame 39 {
              n164 = global write "Globali.vi" "Messaggi"(w441) -> ()
            }
            frame 40 {
              n165 = global write "Globali.vi" "Segnalazioni"(w442) -> ()
            }
            frame 41 {
              n166 = global write "Globali.vi" "Allarmi"(w443) -> ()
            }
            frame 42 {
            }
            frame 43 {
              n167 = Number To Boolean Array(number=w468) -> (Boolean array=w467:bool[])
              n168 = Rotate 1D Array(1:w467, 2:w444) -> (0:w445:bool[])
              n169 = Index Array(array=w445, index #1=0 ("index"), index #2=1 ("index"), index #3=2 ("index"), index #4=3 ("index"), index #5=4 ("index"), index #6=5 ("index"), index #7=6 ("index"), index #8=7 ("index"), index #9=8 ("index"), index #10=9 ("index"), index #11=10 ("index"), index #12=11 ("index"), index #13=12 ("index"), index #14=13 ("index"), index #15=14 ("index"), index #16=15 ("index")) -> (element #1=w450:bool, element #2=w449:bool, element #3=w448:bool, element #4=w447:bool, element #5=w446:bool)  [unwired: 11 out]
              n170 = global write "Globali.vi" "mA_PRESS_INSERZ_ASSE_OK"(w448) -> ()
              n171 = global write "Globali.vi" "mA_TRAZIONE_DISINSERITA"(w446) -> ()
              n172 = global write "Globali.vi" "mA_RISCALDAMENTO_OK"(w449) -> ()
              n173 = global write "Globali.vi" "mA_TRAZIONE_INSERITA"(w447) -> ()
              n174 = global write "Globali.vi" "mA_RICIRCOLO_OK"(w450) -> ()
            }
            frame 44 {
              n175 = Increment(x=w472) -> (x+1=w473:i32)
              n176 = Index Array(array=w474, index=w473) -> (element=w471:u16)
              n177 = call "Double_word_to_real_float.vi"("Seconda WORD"=w471, "Prima WORD"=w470) -> ("Real float"=w469:dbl)  [unwired: 9 in]
              n178 = global write "Globali.vi" "V_TEMP_OLIO_ROD"(w469) -> ()
            }
            frame 45 {
            }
            frame 46 {
              n179 = Number To Boolean Array(number=w495) -> (Boolean array=w494:bool[])
              n180 = Rotate 1D Array(1:w494, 2:w475) -> (0:w476:bool[])
              n181 = Index Array(array=w476, index #1=0 ("index"), index #2=1 ("index"), index #3=2 ("index"), index #4=3 ("index"), index #5=4 ("index"), index #6=5 ("index"), index #7=6 ("index"), index #8=7 ("index"), index #9=8 ("index"), index #10=9 ("index"), index #11=10 ("index"), index #12=11 ("index"), index #13=12 ("index"), index #14=13 ("index"), index #15=14 ("index"), index #16=15 ("index")) -> (element #1=w477:bool)  [unwired: 15 out]
              n182 = global write "Globali.vi" "mA_RODAGGIO_OK"(w477) -> ()
            }
            frame 47 {
              n183 = Increment(x=w499) -> (x+1=w500:i32)
              n184 = Index Array(array=w501, index=w500) -> (element=w498:u16)
              n185 = call "Double_word_to_real_float.vi"("Seconda WORD"=w498, "Prima WORD"=w497) -> ("Real float"=w496:dbl)  [unwired: 9 in]
              n186 = global write "Globali.vi" "V_TEMP_OLIO_1_FUN"(w496) -> ()
            }
            frame 48 {
            }
            frame 49 {
              n187 = Increment(x=w505) -> (x+1=w506:i32)
              n188 = Index Array(array=w507, index=w506) -> (element=w504:u16)
              n189 = call "Double_word_to_real_float.vi"("Seconda WORD"=w504, "Prima WORD"=w503) -> ("Real float"=w502:dbl)  [unwired: 9 in]
              n190 = global write "Globali.vi" "V_COPPIA_1_FUN"(w502) -> ()
            }
            frame 50 {
            }
            frame 51 {
              n191 = Number To Boolean Array(number=w528) -> (Boolean array=w527:bool[])
              n192 = Rotate 1D Array(1:w527, 2:w508) -> (0:w509:bool[])
              n193 = Index Array(array=w509, index #1=0 ("index"), index #2=1 ("index"), index #3=2 ("index"), index #4=3 ("index"), index #5=4 ("index"), index #6=5 ("index"), index #7=6 ("index"), index #8=7 ("index"), index #9=8 ("index"), index #10=9 ("index"), index #11=10 ("index"), index #12=11 ("index"), index #13=12 ("index"), index #14=13 ("index"), index #15=14 ("index"), index #16=15 ("index")) -> (element #1=w510:bool)  [unwired: 15 out]
              n194 = global write "Globali.vi" "mA_COPPIA_1_FUN_OK"(w510) -> ()
            }
            frame 52 {
              n195 = Increment(x=w532) -> (x+1=w533:i32)
              n196 = Index Array(array=w534, index=w533) -> (element=w531:u16)
              n197 = call "Double_word_to_real_float.vi"("Seconda WORD"=w531, "Prima WORD"=w530) -> ("Real float"=w529:dbl)  [unwired: 9 in]
              n198 = global write "Globali.vi" "V_TEMP_CUSCIN_1_FUN_AAT"(w529) -> ()
            }
            frame 53 {
            }
            frame 54 {
              n199 = Increment(x=w538) -> (x+1=w539:i32)
              n200 = Index Array(array=w540, index=w539) -> (element=w537:u16)
              n201 = call "Double_word_to_real_float.vi"("Seconda WORD"=w537, "Prima WORD"=w536) -> ("Real float"=w535:dbl)  [unwired: 9 in]
              n202 = global write "Globali.vi" "V_PRES_OLIO_RICIRC_1_FUN"(w535) -> ()
            }
            frame 55 {
            }
            frame 56 {
              n203 = Number To Boolean Array(number=w561) -> (Boolean array=w560:bool[])
              n204 = Rotate 1D Array(1:w560, 2:w541) -> (0:w542:bool[])
              n205 = Index Array(array=w542, index #1=0 ("index"), index #2=1 ("index"), index #3=2 ("index"), index #4=3 ("index"), index #5=4 ("index"), index #6=5 ("index"), index #7=6 ("index"), index #8=7 ("index"), index #9=8 ("index"), index #10=9 ("index"), index #11=10 ("index"), index #12=11 ("index"), index #13=12 ("index"), index #14=13 ("index"), index #15=14 ("index"), index #16=15 ("index")) -> (element #1=w543:bool)  [unwired: 15 out]
              n206 = global write "Globali.vi" "mA_RICIRCOLO_1_FUN_OK"(w543) -> ()
            }
            frame 57 {
              n207 = Increment(x=w565) -> (x+1=w566:i32)
              n208 = Index Array(array=w567, index=w566) -> (element=w564:u16)
              n209 = call "Double_word_to_real_float.vi"("Seconda WORD"=w564, "Prima WORD"=w563) -> ("Real float"=w562:dbl)  [unwired: 9 in]
              n210 = global write "Globali.vi" "V_PORT_RICIRC_1_FUN_AAT2"(w562) -> ()
            }
            frame 58 {
            }
            frame 59 {
              n211 = Increment(x=w571) -> (x+1=w572:i32)
              n212 = Index Array(array=w573, index=w572) -> (element=w570:u16)
              n213 = call "Double_word_to_real_float.vi"("Seconda WORD"=w570, "Prima WORD"=w569) -> ("Real float"=w568:dbl)  [unwired: 9 in]
              n214 = global write "Globali.vi" "V_TEMP_OLIO_2_FUN"(w568) -> ()
            }
            frame 60 {
            }
            frame 61 {
              n215 = Increment(x=w577) -> (x+1=w578:i32)
              n216 = Index Array(array=w579, index=w578) -> (element=w576:u16)
              n217 = call "Double_word_to_real_float.vi"("Seconda WORD"=w576, "Prima WORD"=w575) -> ("Real float"=w574:dbl)  [unwired: 9 in]
              n218 = global write "Globali.vi" "V_COPPIA_2_FUN"(w574) -> ()
            }
            frame 62 {
            }
            frame 63 {
              n219 = Number To Boolean Array(number=w600) -> (Boolean array=w599:bool[])
              n220 = Rotate 1D Array(1:w599, 2:w580) -> (0:w581:bool[])
              n221 = Index Array(array=w581, index #1=0 ("index"), index #2=1 ("index"), index #3=2 ("index"), index #4=3 ("index"), index #5=4 ("index"), index #6=5 ("index"), index #7=6 ("index"), index #8=7 ("index"), index #9=8 ("index"), index #10=9 ("index"), index #11=10 ("index"), index #12=11 ("index"), index #13=12 ("index"), index #14=13 ("index"), index #15=14 ("index"), index #16=15 ("index")) -> (element #1=w582:bool)  [unwired: 15 out]
              n222 = global write "Globali.vi" "mA_COPPIA_2_FUN_OK"(w582) -> ()
            }
            frame 64 {
              n223 = Increment(x=w604) -> (x+1=w605:i32)
              n224 = Index Array(array=w606, index=w605) -> (element=w603:u16)
              n225 = call "Double_word_to_real_float.vi"("Seconda WORD"=w603, "Prima WORD"=w602) -> ("Real float"=w601:dbl)  [unwired: 9 in]
              n226 = global write "Globali.vi" "V_TEMP_CUSCIN_2_FUN_AAT"(w601) -> ()
            }
            frame 65 {
            }
            frame 66 {
              n227 = Increment(x=w610) -> (x+1=w611:i32)
              n228 = Index Array(array=w612, index=w611) -> (element=w609:u16)
              n229 = call "Double_word_to_real_float.vi"("Seconda WORD"=w609, "Prima WORD"=w608) -> ("Real float"=w607:dbl)  [unwired: 9 in]
              n230 = global write "Globali.vi" "V_PRES_OLIO_RICIRC_2_FUN"(w607) -> ()
            }
            frame 67 {
            }
            frame 68 {
              n231 = Number To Boolean Array(number=w633) -> (Boolean array=w632:bool[])
              n232 = Rotate 1D Array(1:w632, 2:w613) -> (0:w614:bool[])
              n233 = Index Array(array=w614, index #1=0 ("index"), index #2=1 ("index"), index #3=2 ("index"), index #4=3 ("index"), index #5=4 ("index"), index #6=5 ("index"), index #7=6 ("index"), index #8=7 ("index"), index #9=8 ("index"), index #10=9 ("index"), index #11=10 ("index"), index #12=11 ("index"), index #13=12 ("index"), index #14=13 ("index"), index #15=14 ("index"), index #16=15 ("index")) -> (element #1=w615:bool)  [unwired: 15 out]
              n234 = global write "Globali.vi" "mA_RICIRCOLO_2_FUN_OK"(w615) -> ()
            }
            frame 69 {
              n235 = Increment(x=w637) -> (x+1=w638:i32)
              n236 = Index Array(array=w639, index=w638) -> (element=w636:u16)
              n237 = call "Double_word_to_real_float.vi"("Seconda WORD"=w636, "Prima WORD"=w635) -> ("Real float"=w634:dbl)  [unwired: 9 in]
              n238 = global write "Globali.vi" "V_PORT_RICIRC_2_FUN_AAT2"(w634) -> ()
            }
            frame 70 {
            }
            frame 71 {
              n239 = Increment(x=w643) -> (x+1=w644:i32)
              n240 = Index Array(array=w645, index=w644) -> (element=w642:u16)
              n241 = call "Double_word_to_real_float.vi"("Seconda WORD"=w642, "Prima WORD"=w641) -> ("Real float"=w640:dbl)  [unwired: 9 in]
              n242 = global write "Globali.vi" "V_TEMP_OLIO_3_FUN"(w640) -> ()
            }
            frame 72 {
            }
            frame 73 {
              n243 = Increment(x=w649) -> (x+1=w650:i32)
              n244 = Index Array(array=w651, index=w650) -> (element=w648:u16)
              n245 = call "Double_word_to_real_float.vi"("Seconda WORD"=w648, "Prima WORD"=w647) -> ("Real float"=w646:dbl)  [unwired: 9 in]
              n246 = global write "Globali.vi" "V_COPPIA_3_FUN"(w646) -> ()
            }
            frame 74 {
            }
            frame 75 {
              n247 = Number To Boolean Array(number=w672) -> (Boolean array=w671:bool[])
              n248 = Rotate 1D Array(1:w671, 2:w652) -> (0:w653:bool[])
              n249 = Index Array(array=w653, index #1=0 ("index"), index #2=1 ("index"), index #3=2 ("index"), index #4=3 ("index"), index #5=4 ("index"), index #6=5 ("index"), index #7=6 ("index"), index #8=7 ("index"), index #9=8 ("index"), index #10=9 ("index"), index #11=10 ("index"), index #12=11 ("index"), index #13=12 ("index"), index #14=13 ("index"), index #15=14 ("index"), index #16=15 ("index")) -> (element #1=w654:bool)  [unwired: 15 out]
              n250 = global write "Globali.vi" "mA_COPPIA_3_FUN_OK"(w654) -> ()
            }
            frame 76 {
              n251 = Increment(x=w676) -> (x+1=w677:i32)
              n252 = Index Array(array=w678, index=w677) -> (element=w675:u16)
              n253 = call "Double_word_to_real_float.vi"("Seconda WORD"=w675, "Prima WORD"=w674) -> ("Real float"=w673:dbl)  [unwired: 9 in]
              n254 = global write "Globali.vi" "V_TEMP_CUSCIN_3_FUN_AAT"(w673) -> ()
            }
            frame 77 {
            }
            frame 78 {
              n255 = Increment(x=w682) -> (x+1=w683:i32)
              n256 = Index Array(array=w684, index=w683) -> (element=w681:u16)
              n257 = call "Double_word_to_real_float.vi"("Seconda WORD"=w681, "Prima WORD"=w680) -> ("Real float"=w679:dbl)  [unwired: 9 in]
              n258 = global write "Globali.vi" "V_PRES_OLIO_RICIRC_3_FUN"(w679) -> ()
            }
            frame 79 {
            }
            frame 80 {
              n259 = Number To Boolean Array(number=w705) -> (Boolean array=w704:bool[])
              n260 = Rotate 1D Array(1:w704, 2:w685) -> (0:w686:bool[])
              n261 = Index Array(array=w686, index #1=0 ("index"), index #2=1 ("index"), index #3=2 ("index"), index #4=3 ("index"), index #5=4 ("index"), index #6=5 ("index"), index #7=6 ("index"), index #8=7 ("index"), index #9=8 ("index"), index #10=9 ("index"), index #11=10 ("index"), index #12=11 ("index"), index #13=12 ("index"), index #14=13 ("index"), index #15=14 ("index"), index #16=15 ("index")) -> (element #1=w687:bool)  [unwired: 15 out]
              n262 = global write "Globali.vi" "mA_RICIRCOLO_3_FUN_OK"(w687) -> ()
            }
            frame 81 {
              n263 = Increment(x=w709) -> (x+1=w710:i32)
              n264 = Index Array(array=w711, index=w710) -> (element=w708:u16)
              n265 = call "Double_word_to_real_float.vi"("Seconda WORD"=w708, "Prima WORD"=w707) -> ("Real float"=w706:dbl)  [unwired: 9 in]
              n266 = global write "Globali.vi" "V_PORT_RICIRC_3_FUN_AAT2"(w706) -> ()
            }
            frame 82 {
            }
            frame 83 {
              n267 = Number To Boolean Array(number=w734) -> (Boolean array=w733:bool[])
              n268 = Rotate 1D Array(1:w733, 2:w712) -> (0:w713:bool[])
              n269 = Index Array(array=w713, index #1=0 ("index"), index #2=1 ("index"), index #3=2 ("index"), index #4=3 ("index"), index #5=4 ("index"), index #6=5 ("index"), index #7=6 ("index"), index #8=7 ("index"), index #9=8 ("index"), index #10=9 ("index"), index #11=10 ("index"), index #12=11 ("index"), index #13=12 ("index"), index #14=13 ("index"), index #15=14 ("index"), index #16=15 ("index")) -> (element #1=w716:bool, element #2=w715:bool, element #3=w714:bool)  [unwired: 13 out]
              n270 = global write "Globali.vi" "mA_GONFIAGGIO_OK"(w716) -> ()
              n271 = global write "Globali.vi" "mA_PERDITE_DX_OK"(w715) -> ()
              n272 = global write "Globali.vi" "mA_PERDITE_SX_OK"(w714) -> ()
            }
            frame 84 {
              n273 = Increment(x=w738) -> (x+1=w739:i32)
              n274 = Index Array(array=w740, index=w739) -> (element=w737:u16)
              n275 = call "Double_word_to_real_float.vi"("Seconda WORD"=w737, "Prima WORD"=w736) -> ("Real float"=w735:dbl)  [unwired: 9 in]
              n276 = global write "Globali.vi" "V_TEMP_OLIO_4_FUN"(w735) -> ()
            }
            frame 85 {
            }
            frame 86 {
              n277 = Increment(x=w744) -> (x+1=w745:i32)
              n278 = Index Array(array=w746, index=w745) -> (element=w743:u16)
              n279 = call "Double_word_to_real_float.vi"("Seconda WORD"=w743, "Prima WORD"=w742) -> ("Real float"=w741:dbl)  [unwired: 9 in]
              n280 = global write "Globali.vi" "V_COPPIA_4_FUN"(w741) -> ()
            }
            frame 87 {
            }
            frame 88 {
              n281 = Number To Boolean Array(number=w767) -> (Boolean array=w766:bool[])
              n282 = Rotate 1D Array(1:w766, 2:w747) -> (0:w748:bool[])
              n283 = Index Array(array=w748, index #1=0 ("index"), index #2=1 ("index"), index #3=2 ("index"), index #4=3 ("index"), index #5=4 ("index"), index #6=5 ("index"), index #7=6 ("index"), index #8=7 ("index"), index #9=8 ("index"), index #10=9 ("index"), index #11=10 ("index"), index #12=11 ("index"), index #13=12 ("index"), index #14=13 ("index"), index #15=14 ("index"), index #16=15 ("index")) -> (element #1=w749:bool)  [unwired: 15 out]
              n284 = global write "Globali.vi" "mA_COPPIA_4_FUN_OK"(w749) -> ()
            }
            frame 89 {
              n285 = Increment(x=w771) -> (x+1=w772:i32)
              n286 = Index Array(array=w773, index=w772) -> (element=w770:u16)
              n287 = call "Double_word_to_real_float.vi"("Seconda WORD"=w770, "Prima WORD"=w769) -> ("Real float"=w768:dbl)  [unwired: 9 in]
              n288 = global write "Globali.vi" "V_TEMP_CUSCIN_4_FUN_AAT"(w768) -> ()
            }
            frame 90 {
            }
            frame 91 {
              n289 = Increment(x=w777) -> (x+1=w778:i32)
              n290 = Index Array(array=w779, index=w778) -> (element=w776:u16)
              n291 = call "Double_word_to_real_float.vi"("Seconda WORD"=w776, "Prima WORD"=w775) -> ("Real float"=w774:dbl)  [unwired: 9 in]
              n292 = global write "Globali.vi" "V_PRES_OLIO_RICIRC_4_FUN"(w774) -> ()
            }
            frame 92 {
            }
            frame 93 {
              n293 = Number To Boolean Array(number=w800) -> (Boolean array=w799:bool[])
              n294 = Rotate 1D Array(1:w799, 2:w780) -> (0:w781:bool[])
              n295 = Index Array(array=w781, index #1=0 ("index"), index #2=1 ("index"), index #3=2 ("index"), index #4=3 ("index"), index #5=4 ("index"), index #6=5 ("index"), index #7=6 ("index"), index #8=7 ("index"), index #9=8 ("index"), index #10=9 ("index"), index #11=10 ("index"), index #12=11 ("index"), index #13=12 ("index"), index #14=13 ("index"), index #15=14 ("index"), index #16=15 ("index")) -> (element #1=w782:bool)  [unwired: 15 out]
              n296 = global write "Globali.vi" "mA_RICIRCOLO_4_FUN_OK"(w782) -> ()
            }
            frame 94 {
              n297 = Increment(x=w804) -> (x+1=w805:i32)
              n298 = Index Array(array=w806, index=w805) -> (element=w803:u16)
              n299 = call "Double_word_to_real_float.vi"("Seconda WORD"=w803, "Prima WORD"=w802) -> ("Real float"=w801:dbl)  [unwired: 9 in]
              n300 = global write "Globali.vi" "V_PORT_RICIRC_4_FUN_AAT2"(w801) -> ()
            }
            frame 95 {
            }
            frame 96 {
              n301 = Increment(x=w810) -> (x+1=w811:i32)
              n302 = Index Array(array=w812, index=w811) -> (element=w809:u16)
              n303 = call "Double_word_to_real_float.vi"("Seconda WORD"=w809, "Prima WORD"=w808) -> ("Real float"=w807:dbl)  [unwired: 9 in]
              n304 = global write "Globali.vi" "V_TEMP_OLIO_5_FUN"(w807) -> ()
            }
            frame 97 {
            }
            frame 98 {
              n305 = Increment(x=w816) -> (x+1=w817:i32)
              n306 = Index Array(array=w818, index=w817) -> (element=w815:u16)
              n307 = call "Double_word_to_real_float.vi"("Seconda WORD"=w815, "Prima WORD"=w814) -> ("Real float"=w813:dbl)  [unwired: 9 in]
              n308 = global write "Globali.vi" "V_COPPIA_5_FUN"(w813) -> ()
            }
            frame 99 {
            }
            frame 100 {
              n309 = Number To Boolean Array(number=w839) -> (Boolean array=w838:bool[])
              n310 = Rotate 1D Array(1:w838, 2:w819) -> (0:w820:bool[])
              n311 = Index Array(array=w820, index #1=0 ("index"), index #2=1 ("index"), index #3=2 ("index"), index #4=3 ("index"), index #5=4 ("index"), index #6=5 ("index"), index #7=6 ("index"), index #8=7 ("index"), index #9=8 ("index"), index #10=9 ("index"), index #11=10 ("index"), index #12=11 ("index"), index #13=12 ("index"), index #14=13 ("index"), index #15=14 ("index"), index #16=15 ("index")) -> (element #1=w821:bool)  [unwired: 15 out]
              n312 = global write "Globali.vi" "mA_COPPIA_5_FUN_OK"(w821) -> ()
            }
            frame 101 {
              n313 = Increment(x=w843) -> (x+1=w844:i32)
              n314 = Index Array(array=w845, index=w844) -> (element=w842:u16)
              n315 = call "Double_word_to_real_float.vi"("Seconda WORD"=w842, "Prima WORD"=w841) -> ("Real float"=w840:dbl)  [unwired: 9 in]
              n316 = global write "Globali.vi" "V_TEMP_CUSCIN_5_FUN_AAT"(w840) -> ()
            }
            frame 102 {
            }
            frame 103 {
              n317 = Increment(x=w849) -> (x+1=w850:i32)
              n318 = Index Array(array=w851, index=w850) -> (element=w848:u16)
              n319 = call "Double_word_to_real_float.vi"("Seconda WORD"=w848, "Prima WORD"=w847) -> ("Real float"=w846:dbl)  [unwired: 9 in]
              n320 = global write "Globali.vi" "V_PRES_OLIO_RICIRC_5_FUN"(w846) -> ()
            }
            frame 104 {
            }
            frame 105 {
              n321 = Number To Boolean Array(number=w872) -> (Boolean array=w871:bool[])
              n322 = Rotate 1D Array(1:w871, 2:w852) -> (0:w853:bool[])
              n323 = Index Array(array=w853, index #1=0 ("index"), index #2=1 ("index"), index #3=2 ("index"), index #4=3 ("index"), index #5=4 ("index"), index #6=5 ("index"), index #7=6 ("index"), index #8=7 ("index"), index #9=8 ("index"), index #10=9 ("index"), index #11=10 ("index"), index #12=11 ("index"), index #13=12 ("index"), index #14=13 ("index"), index #15=14 ("index"), index #16=15 ("index")) -> (element #1=w854:bool)  [unwired: 15 out]
              n324 = global write "Globali.vi" "mA_RICIRCOLO_5_FUN_OK"(w854) -> ()
            }
            frame 106 {
              n325 = Increment(x=w876) -> (x+1=w877:i32)
              n326 = Index Array(array=w878, index=w877) -> (element=w875:u16)
              n327 = call "Double_word_to_real_float.vi"("Seconda WORD"=w875, "Prima WORD"=w874) -> ("Real float"=w873:dbl)  [unwired: 9 in]
              n328 = global write "Globali.vi" "V_PORT_RICIRC_5_FUN_AAT2"(w873) -> ()
            }
            frame 107 {
            }
            frame 108 {
              n329 = Number To Boolean Array(number=w899) -> (Boolean array=w898:bool[])
              n330 = Rotate 1D Array(1:w898, 2:w879) -> (0:w880:bool[])
              n331 = Index Array(array=w880, index #1=0 ("index"), index #2=1 ("index"), index #3=2 ("index"), index #4=3 ("index"), index #5=4 ("index"), index #6=5 ("index"), index #7=6 ("index"), index #8=7 ("index"), index #9=8 ("index"), index #10=9 ("index"), index #11=10 ("index"), index #12=11 ("index"), index #13=12 ("index"), index #14=13 ("index"), index #15=14 ("index"), index #16=15 ("index")) -> (element #1=w881:bool)  [unwired: 15 out]
              n332 = global write "Globali.vi" "mA_PRESS_PRESSURIZZ_OK"(w881) -> ()
            }
            frame 109 {
              n333 = Increment(x=w903) -> (x+1=w904:i32)
              n334 = Index Array(array=w905, index=w904) -> (element=w902:u16)
              n335 = call "Double_word_to_real_float.vi"("Seconda WORD"=w902, "Prima WORD"=w901) -> ("Real float"=w900:dbl)  [unwired: 9 in]
              n336 = global write "Globali.vi" "V_PRESS_PRESSURIZZ"(w900) -> ()
            }
            frame 110 {
            }
            frame 111 {
              n337 = Number To Boolean Array(number=w927) -> (Boolean array=w926:bool[])
              n338 = Rotate 1D Array(1:w926, 2:w906) -> (0:w907:bool[])
              n339 = Index Array(array=w907, index #1=0 ("index"), index #2=1 ("index"), index #3=2 ("index"), index #4=3 ("index"), index #5=4 ("index"), index #6=5 ("index"), index #7=6 ("index"), index #8=7 ("index"), index #9=8 ("index"), index #10=9 ("index"), index #11=10 ("index"), index #12=11 ("index"), index #13=12 ("index"), index #14=13 ("index"), index #15=14 ("index"), index #16=15 ("index")) -> (element #1=w909:bool, element #2=w908:bool)  [unwired: 14 out]
              n340 = global write "Globali.vi" "mA_PRESSURIZZ_DX_OK"(w909) -> ()
              n341 = global write "Globali.vi" "mA_PRESSURIZZ_SX_OK"(w908) -> ()
            }
            frame 112 {
              n342 = Increment(x=w930) -> (x+1=w933:i32)
              n343 = Index Array(array=w929, index=w933) -> (element=w932:u16)
              n344 = call "Double_word_to_real_float.vi"("Seconda WORD"=w932, "Prima WORD"=w928) -> ("Real float"=w931:dbl)  [unwired: 9 in]
              n345 = global write "Globali.vi" "V_PERDITA_GONFIAGGIO_DX"(w931) -> ()
            }
            frame 113 {
            }
            frame 114 {
              n346 = Increment(x=w934) -> (x+1=w939:i32)
              n347 = Index Array(array=w935, index=w939) -> (element=w938:u16)
              n348 = call "Double_word_to_real_float.vi"("Seconda WORD"=w938, "Prima WORD"=w936) -> ("Real float"=w937:dbl)  [unwired: 9 in]
              n349 = global write "Globali.vi" "V_PERDITA_GONFIAGGIO_SX"(w937) -> ()
            }
            frame 115 {
            }
            frame 116 {
              n350 = Increment(x=w940) -> (x+1=w945:i32)
              n351 = Index Array(array=w941, index=w945) -> (element=w944:u16)
              n352 = call "Double_word_to_real_float.vi"("Seconda WORD"=w944, "Prima WORD"=w942) -> ("Real float"=w943:dbl)  [unwired: 9 in]
              n353 = global write "Globali.vi" "V_PERDITA_PRESSURIZZ_DX"(w943) -> ()
            }
            frame 117 {
            }
            frame 118 {
              n354 = Increment(x=w946) -> (x+1=w951:i32)
              n355 = Index Array(array=w947, index=w951) -> (element=w950:u16)
              n356 = call "Double_word_to_real_float.vi"("Seconda WORD"=w950, "Prima WORD"=w948) -> ("Real float"=w949:dbl)  [unwired: 9 in]
              n357 = global write "Globali.vi" "V_PERDITA_PRESSURIZZ_SX"(w949) -> ()
            }
            frame 119 {
            }
            frame 120 {
              n358 = Increment(x=w952) -> (x+1=w957:i32)
              n359 = Index Array(array=w953, index=w957) -> (element=w956:u16)
              n360 = call "Double_word_to_real_float.vi"("Seconda WORD"=w956, "Prima WORD"=w954) -> ("Real float"=w955:dbl)  [unwired: 9 in]
              n361 = global write "Globali.vi" "V_SOVRAPRESSIONE_DX"(w955) -> ()
            }
            frame 121 {
            }
            frame 122 {
              n362 = Increment(x=w958) -> (x+1=w963:i32)
              n363 = Index Array(array=w959, index=w963) -> (element=w962:u16)
              n364 = call "Double_word_to_real_float.vi"("Seconda WORD"=w962, "Prima WORD"=w960) -> ("Real float"=w961:dbl)  [unwired: 9 in]
              n365 = global write "Globali.vi" "V_SOVRAPRESSIONE_SX"(w961) -> ()
            }
            frame 123 {
            }
            frame 124 {
              n366 = Number To Boolean Array(number=w968) -> (Boolean array=w987:bool[])
              n367 = Rotate 1D Array(1:w987, 2:w967) -> (0:w969:bool[])
              n368 = Index Array(array=w969, index #1=0 ("index"), index #2=1 ("index"), index #3=2 ("index"), index #4=3 ("index"), index #5=4 ("index"), index #6=5 ("index"), index #7=6 ("index"), index #8=7 ("index"), index #9=8 ("index"), index #10=9 ("index"), index #11=10 ("index"), index #12=11 ("index"), index #13=12 ("index"), index #14=13 ("index"), index #15=14 ("index"), index #16=15 ("index")) -> (element #1=w970:bool, element #2=w966:bool, element #3=w965:bool, element #4=w964:bool)  [unwired: 12 out]
              n369 = global write "Globali.vi" "CICLO_IN_CORSO"(w965) -> ()
              n370 = global write "Globali.vi" "S_VERNICIATO"(w964) -> ()
              n371 = global write "Globali.vi" "S_SCARTO"(w966) -> ()
              n372 = global write "Globali.vi" "S_PAUSA"(w970) -> ()
            }
            frame 125 {
              n373 = global write "Globali.vi" "Cicli_macchina"(w988) -> ()
            }
            frame 126 {
            }
            frame 127 {
            }
            frame Default {
            }
          }
        }
      }
      frame #3 {
        n374 = Wait Until Next ms Multiple(millisecond multiple=u32 50) -> ()  [unwired: 1 out]
      }
      frame #4 {
        # "Scrivo sulla variabile Fase_collaudo solo dopo che ho aggiornato tutte le altre variabili"
        n375 = global write "Globali.vi" "Fase_collaudo"(w990) -> ()
      }
    }
    n376 = Wait Until Next ms Multiple(millisecond multiple=u32 50) -> ()  [unwired: 1 out]
    n377 = global read "Globali.vi" "stop"() -> (w1:bool)
  }
